vi "MARS_Scan_Data_Analysis_global.vi"() -> ()   [LabVIEW 2015]
panel:
  in  "Channels":string[][](array[string])
  out "Channel names":string[](array[string])
  out "selected path":path
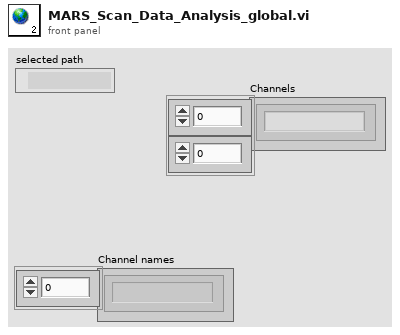
[diagram p1: front panel]
diagram:
